vi "Mix signal measurement_1022D.vi"() -> ()   [LabVIEW 2022 SP3]
uses:
  <vilib>/Analysis/baseanly.llb/Mean (DBL).vi
  <vilib>/Utility/file.llb/Write Delimited Spreadsheet (DBL).vi
  <vilib>/Analysis/NI_AALBase.lvlib
panel:
  out "B Frequency(Hz)":sgl=1000.0 min=0.001 max=100000 step=0.001 format="%.3f"
  out "A Frequency(Hz)":sgl=1000.0 min=0.001 max=100000 step=0.001 format="%.3f"
  in  "Differntial  Frequency":dbl=10267.0 format="%#_13g"
  in  "Base Frequency":dbl=10267.0 format="%#_13g"
  in  "Reference Source":u8(ring) items=["External", "Internal", "Internal Sweep", "Channel A"]
  out "B Sum Frequency":dbl=267.77 format="%#_13g"
  in  "B Input Connection (0: Single-Ended)  2":u16(ring)=1 items=["Single-Ended Voltage", "Differential Voltage", "1 MOhm Current Gain", "100 MOhm Current Gain"]
  in  "B harmonic 4":u8=2
  in  "B harmonic 3":u8=3
  in  "B reference Manual Phase 2":dbl=-59.75
  in  "auto phase B 2":bool=TRUE
  in  "B Sample time (s) 2":dbl=0.001 min=0.001 max=100.0 step=0.001
  in  "B Sensitivity  2":u16(ring)=21 items=["1 nV/fA", "2 nV/fA", "5 nV/fA", "10 nV/fA", "20 nV/fA", "50 nV/fA", "100 nV/fA", "200 nV/fA", "500 nV/fA", "1 uV/pA", "2 uV/pA", "5 uV/pA", "10 uV/pA", "20 uV/pA", "50 uV/pA", "100 uV/pA", "200 uV/pA", "500 uV/pA", "1 mV/nA", "2 mV/nA", "5 mV/nA", "10 mV/nA", "20 mV/nA", "50 mV/nA", "100 mV/nA", "200 mV/nA", "500 mV/nA", "1 V/uA"]
  in  "Enable Sync Filter B (open when f<200Hz) 2":bool
  in  "B Time Constant 2":u8(ring)=9 items=["10 us", "30 us", "100 us", "300 us", "1 ms", "3 ms", "10 ms", "30 ms", "100 ms", "300 ms", "1 s", "3 s", "10 s", "30 s", "100 s", "300 s", "1 ks", "3 ks"]
  in  "B Reference Source 2":u8(ring)=1 items=["External", "Internal", "Internal Sweep", "Channel-A"]
  in  "B Low Pass Filter Slope 2":u8(ring)=2 items=["6 dB/oct", "12 dB/oct", "18 db/oct", "24 dB/oct"]
  out "A  Sub Frequency":dbl=267.77 format="%#_13g"
  in  "A Input Connection (0: Single-Ended)  2":u16(ring)=1 items=["Single-Ended Voltage", "Differential Voltage", "1 MOhm Current Gain", "100 MOhm Current Gain"]
  in  "A harmonic 4":u8=2
  in  "A harmonic 3":u8=3
  in  "A reference Manual Phase  2":dbl=-59.75
  in  "auto phase A 2":bool=TRUE
  in  "A Reference Source 2":u8(ring)=1 items=["External", "Internal", "Internal Sweep"]
  in  "A Sample time (s) 2":dbl=0.001 min=0.001 max=100.0 step=0.001
  in  "A Time Constant 2":u8(ring)=9 items=["10 us", "30 us", "100 us", "300 us", "1 ms", "3 ms", "10 ms", "30 ms", "100 ms", "300 ms", "1 s", "3 s", "10 s", "30 s", "100 s", "300 s", "1 ks", "3 ks"]
  in  "Enable Sync Filter A (open when f<200Hz) 2":bool
  in  "A Sensitivity  2":u16(ring)=21 items=["1 nV/fA", "2 nV/fA", "5 nV/fA", "10 nV/fA", "20 nV/fA", "50 nV/fA", "100 nV/fA", "200 nV/fA", "500 nV/fA", "1 uV/pA", "2 uV/pA", "5 uV/pA", "10 uV/pA", "20 uV/pA", "50 uV/pA", "100 uV/pA", "200 uV/pA", "500 uV/pA", "1 mV/nA", "2 mV/nA", "5 mV/nA", "10 mV/nA", "20 mV/nA", "50 mV/nA", "100 mV/nA", "200 mV/nA", "500 mV/nA", "1 V/uA"]
  in  "A Low Pass Filter Slope 2":u8(ring)=2 items=["6 dB/oct", "12 dB/oct", "18 db/oct", "24 dB/oct"]
  in  "LOCKIN2 address":refnum<visa-resource-name>="COM7"
  in  "Series Resistance":string="20kOhm"
  in  "Temperature \n& Field Function":bool=TRUE
  in  "Field Approach":i32(ring) items=["Linear", "NoOvershoot", "Oscillate"]
  in  "F Rate (Oe/s)":dbl=100.0 format="%#_13g"
  in  "Set F (Oe)":dbl format="%#_13g"
  in  "Mode":i32(ring) items=["Persistent", "Driven"]
  in  "Temperature Approach":i32(ring)=1 items=["FastSettle", "NoOvershoot"]
  in  "T  Rate (K/min)":dbl=10.0
  in  "Set  T  (K)":dbl=120.0
  in  "WaitForField":bool=TRUE
  in  "WaitForTemperature":bool=TRUE
  out "Temperature Status":i32(ring) items=["TemperatureUnknown"=0, "Stable"=1, "Tracking"=2, "Near"=5, "Chasing"=6, "Filling"=7, "Standby"=10, "Disabled"=13, "ImpedanceNotFunction"=14, "TempFailure"=15]
  out "Field Status":i32(ring) items=["MagnetUnknown"=0, "StablePersistent"=1, "WarmingSwitch"=2, "CoolingSwitch"=3, "StableDriven"=4, "Iterating"=5, "Charging"=6, "Discharging"=7, "CurrentError"=8, "MagnetFailure"=15]
  out "Field":dbl
  in  "Delay":dbl=5.0
  out "Temperature":dbl
  in  "Remote":bool=TRUE
  in  "IP Address":string="169.254.170.239"
  out "Measuring":bool
  in  "A Low Pass Filter Slope":u8(ring)=2 items=["6 dB/oct", "12 dB/oct", "18 db/oct", "24 dB/oct"]
  in  "B Low Pass Filter Slope":u8(ring)=2 items=["6 dB/oct", "12 dB/oct", "18 db/oct", "24 dB/oct"]
  in  "B Time Constant":u8(ring)=9 items=["10 us", "30 us", "100 us", "300 us", "1 ms", "3 ms", "10 ms", "30 ms", "100 ms", "300 ms", "1 s", "3 s", "10 s", "30 s", "100 s", "300 s", "1 ks", "3 ks"]
  in  "Enable Sync Filter B (open when f<200Hz)":bool
  in  "B Sensitivity":u16(ring)=23 items=["1 nV/fA", "2 nV/fA", "5 nV/fA", "10 nV/fA", "20 nV/fA", "50 nV/fA", "100 nV/fA", "200 nV/fA", "500 nV/fA", "1 uV/pA", "2 uV/pA", "5 uV/pA", "10 uV/pA", "20 uV/pA", "50 uV/pA", "100 uV/pA", "200 uV/pA", "500 uV/pA", "1 mV/nA", "2 mV/nA", "5 mV/nA", "10 mV/nA", "20 mV/nA", "50 mV/nA", "100 mV/nA", "200 mV/nA", "500 mV/nA", "1 V/uA"]
  in  "A Sensitivity":u16(ring)=23 items=["1 nV/fA", "2 nV/fA", "5 nV/fA", "10 nV/fA", "20 nV/fA", "50 nV/fA", "100 nV/fA", "200 nV/fA", "500 nV/fA", "1 uV/pA", "2 uV/pA", "5 uV/pA", "10 uV/pA", "20 uV/pA", "50 uV/pA", "100 uV/pA", "200 uV/pA", "500 uV/pA", "1 mV/nA", "2 mV/nA", "5 mV/nA", "10 mV/nA", "20 mV/nA", "50 mV/nA", "100 mV/nA", "200 mV/nA", "500 mV/nA", "1 V/uA"]
  in  "Enable Sync Filter A (open when f<200Hz)":bool
  in  "A Time Constant":u8(ring)=9 items=["10 us", "30 us", "100 us", "300 us", "1 ms", "3 ms", "10 ms", "30 ms", "100 ms", "300 ms", "1 s", "3 s", "10 s", "30 s", "100 s", "300 s", "1 ks", "3 ks"]
  out "XY Graph 4":cluster{dbl[], dbl[]}(graph)
  in  "Phase B":u16(ring)=9 items=["X", "Y", "R", "Theta", "Frequency", "Noise", "Xh1", "Yh1", "Rh1", "Theta h1", "Xh2", "Yh2", "Rh2", "Theta h2"]
  in  "Parameter B":u16(ring)=8 items=["X", "Y", "R", "Theta", "Frequency", "Noise", "Xh1", "Yh1", "Rh1", "Theta h1", "Xh2", "Yh2", "Rh2", "Theta h2"]
  out "phase B":dbl
  in  "Clear Plot B":bool
  out "XY Graph 3":cluster{dbl[], dbl[]}(graph)
  out "para2 Measurement":dbl=1.49013e-07
  out "XY Graph 2":cluster{dbl[], dbl[]}(graph)
  in  "B Sample time (s)":dbl=0.001 min=0.001 max=100.0 step=0.001
  in  "A Sample time (s)":dbl=0.001 min=0.001 max=100.0 step=0.001
  in  "Phase A":u16(ring)=9 items=["X", "Y", "R", "Theta", "Frequency", "Noise", "Xh1", "Yh1", "Rh1", "Theta h1", "Xh2", "Yh2", "Rh2", "Theta h2"]
  in  "Parameter A":u16(ring)=8 items=["X", "Y", "R", "Theta", "Frequency", "Noise", "Xh1", "Yh1", "Rh1", "Theta h1", "Xh2", "Yh2", "Rh2", "Theta h2"]
  in  "stabilization(S)":dbl=0.1 format="%#_13g"
  in  "B Input Connection (0: Single-Ended)":u16(ring)=1 items=["Single-Ended Voltage", "Differential Voltage", "1 MOhm Current Gain", "100 MOhm Current Gain"]
  in  "B harmonic 1":u8=2
  in  "B harmonic 2":u8=3
  in  "A Input Connection (0: Single-Ended)":u16(ring)=1 items=["Single-Ended Voltage", "Differential Voltage", "1 MOhm Current Gain", "100 MOhm Current Gain"]
  in  "A harmonic 1":u8=2
  in  "A harmonic 2":u8=3
  in  "A Reference Source":u8(ring)=1 items=["External", "Internal", "Internal Sweep"]
  out "phase A":dbl
  out "loop run":i32
  in  "loop #":i32=1
  in  "Save data or not":bool=TRUE
  in  "path (folder + filename)":string="G:\\My Drive\\Opticool\\Measurement\\NLH\\Signal Mixing\\TaI18_test"
  in  "Clear Plot A":bool
  out "XY Graph":cluster{dbl[], dbl[]}(graph)={[0.18, 0.16, 0.14, 0.12000000000000001, 0.1], [3.3030160227288526e-06, 3.321717991170714e-05, 7.096266610655447e-06, 1.857138617731224e-05, 2.1320792974836174e-05]}
  out "para1 Measurement":dbl=1.49013e-07
  out "Sine voltage":dbl format="%#_13g"
  in  "GATE STEP(mv)":i32=20
  in  "Sine Low Value (default 0V)":dbl=0.1
  in  "Sine High Value (0.001-5V)":dbl=1.0
  in  "lockin waiting (s)":dbl=0.1 format="%#_13g"
  in  "LOCKIN1 address":refnum<visa-resource-name>="COM3"
  # "Lock-in 1 Setting (Input)"
  # "Channel A"
  # "Channel B"
  # "Lock-in 2 Setting (Measure)"
  # "Channel A"
  # "Channel B"
  # "Mesurement"
  # "Sine Sweep Setting"
  # "Temprature and Field Setting"
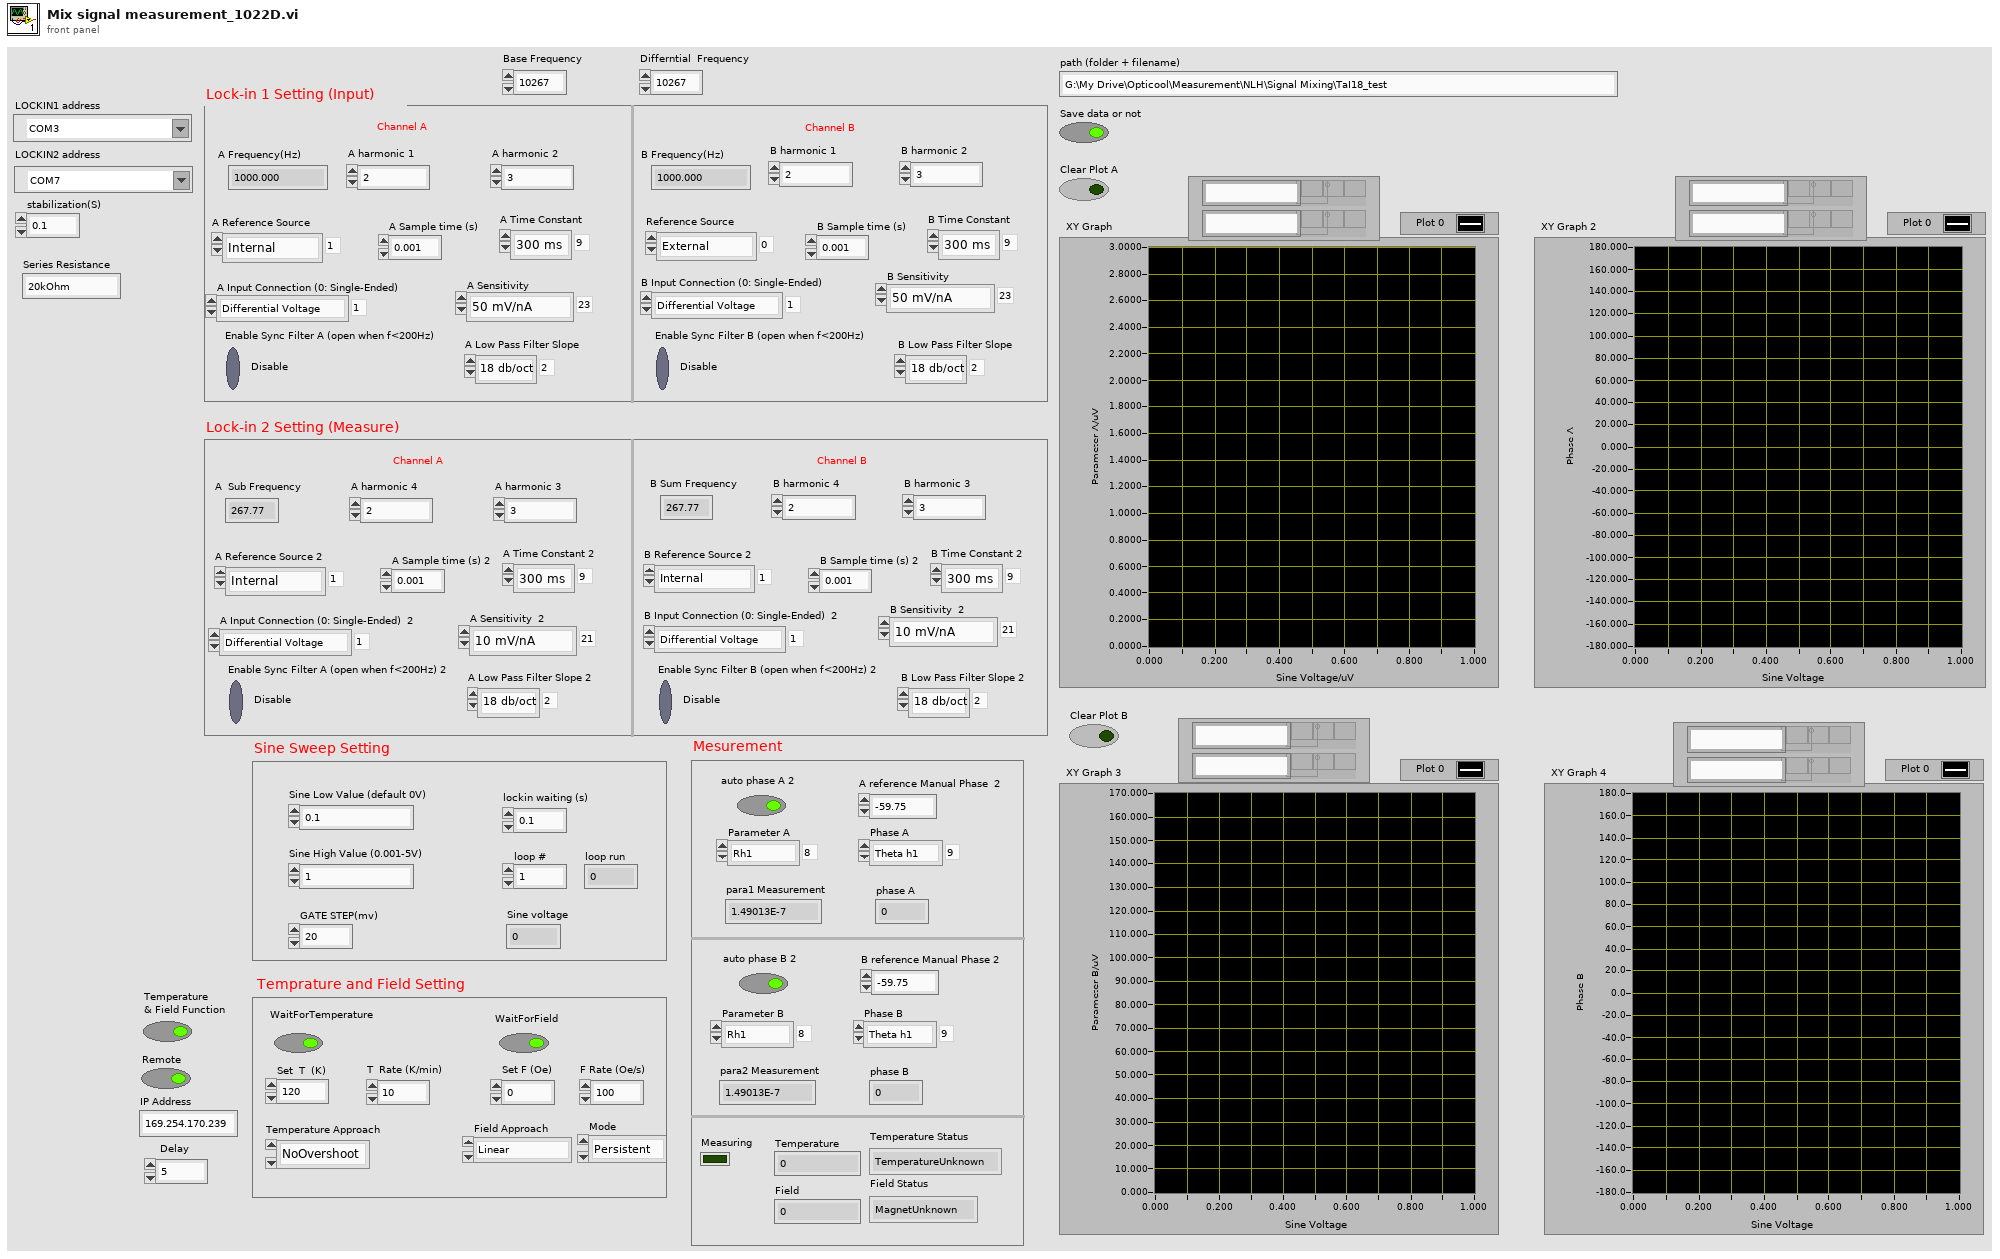
[diagram p1: front panel]
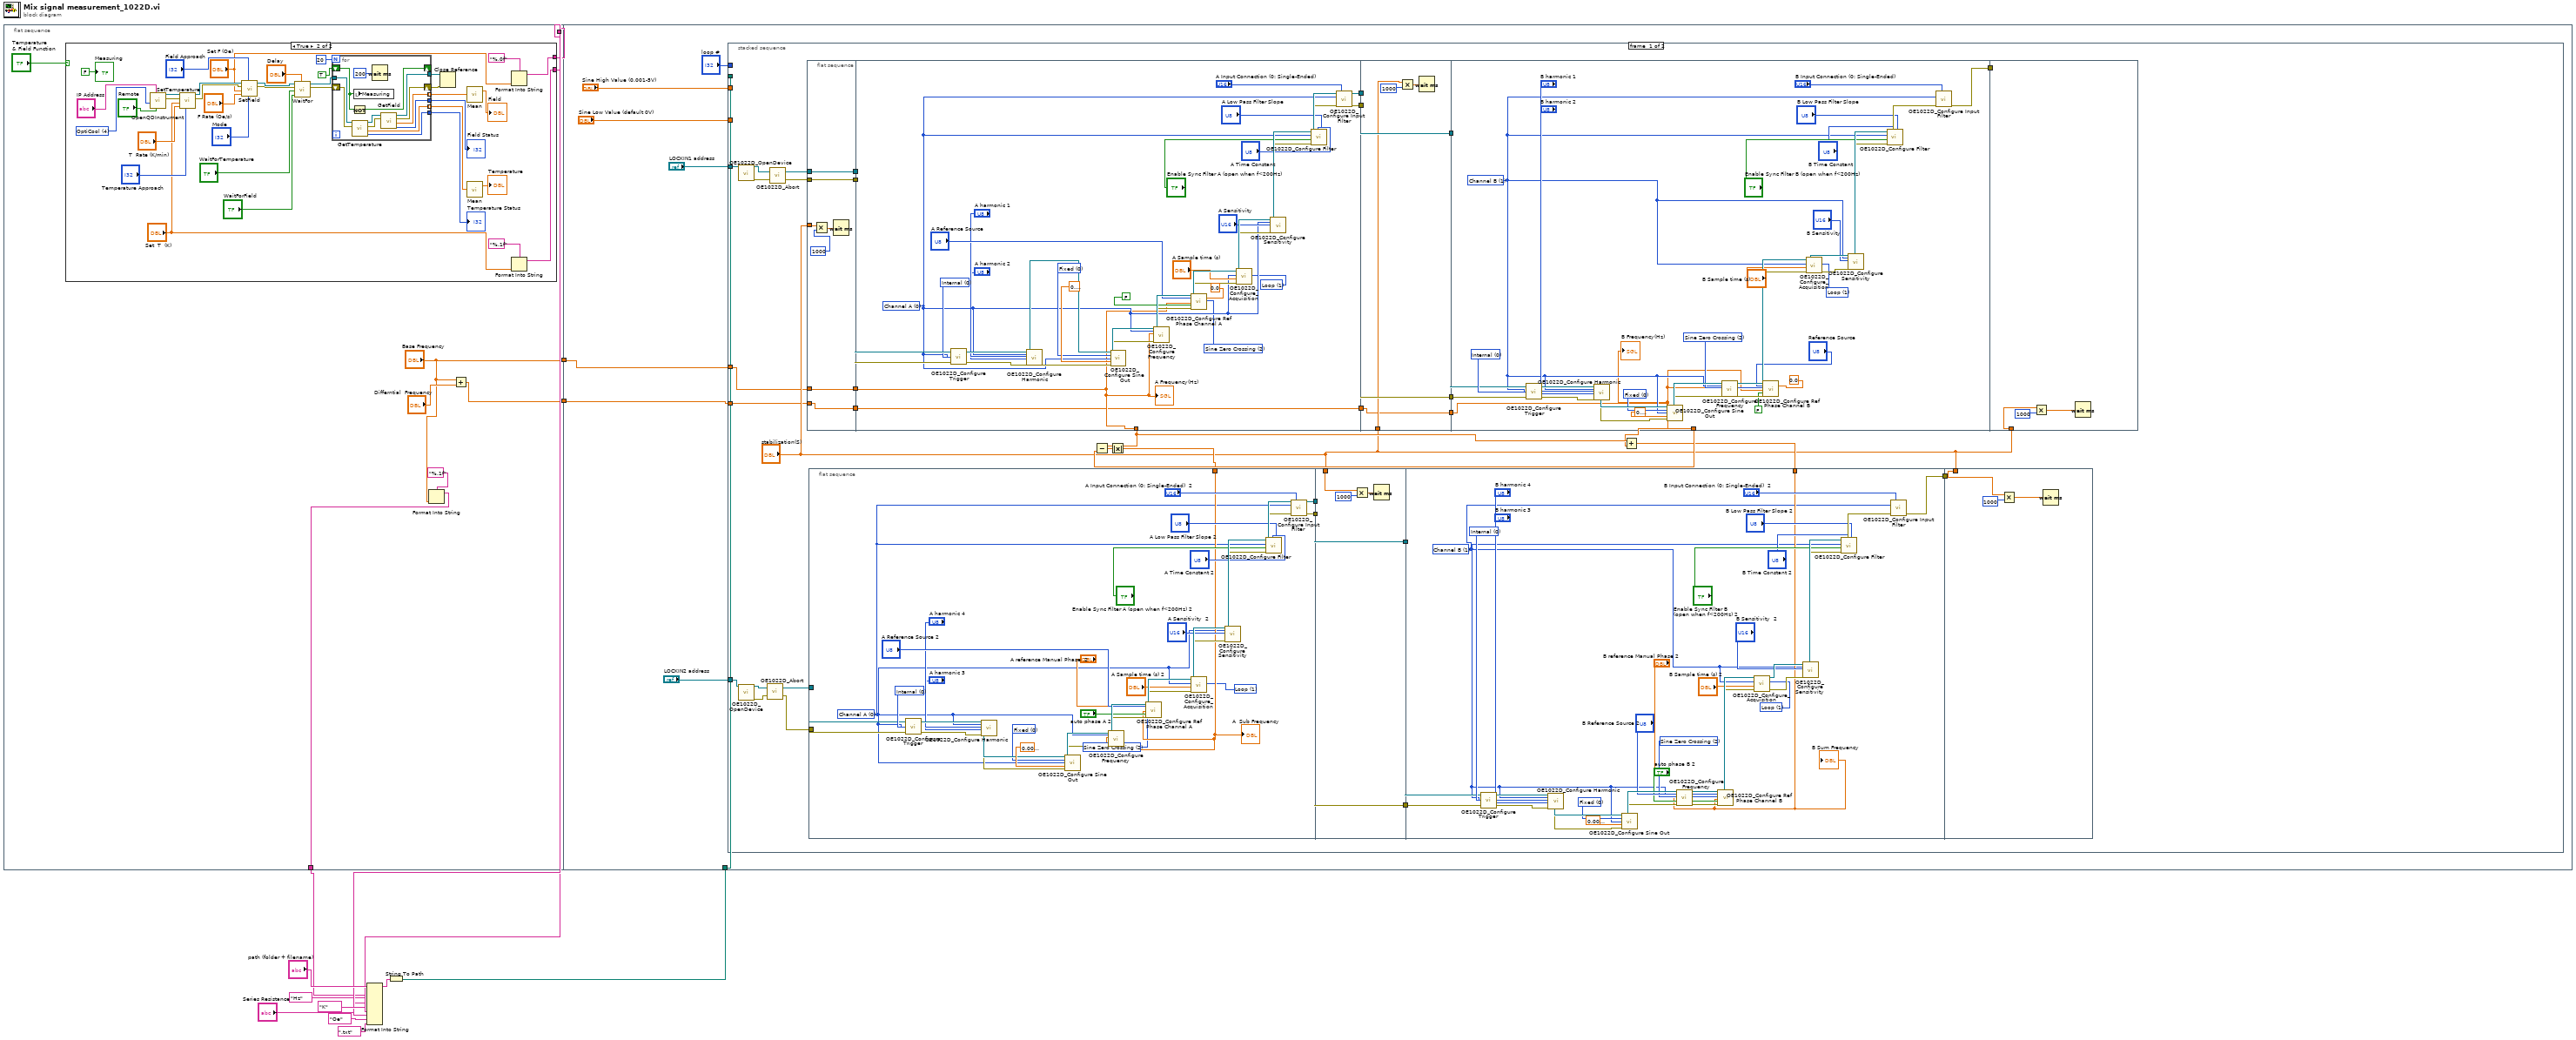
[diagram p0: block diagram]
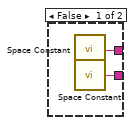
[diagram p2: hidden frame]
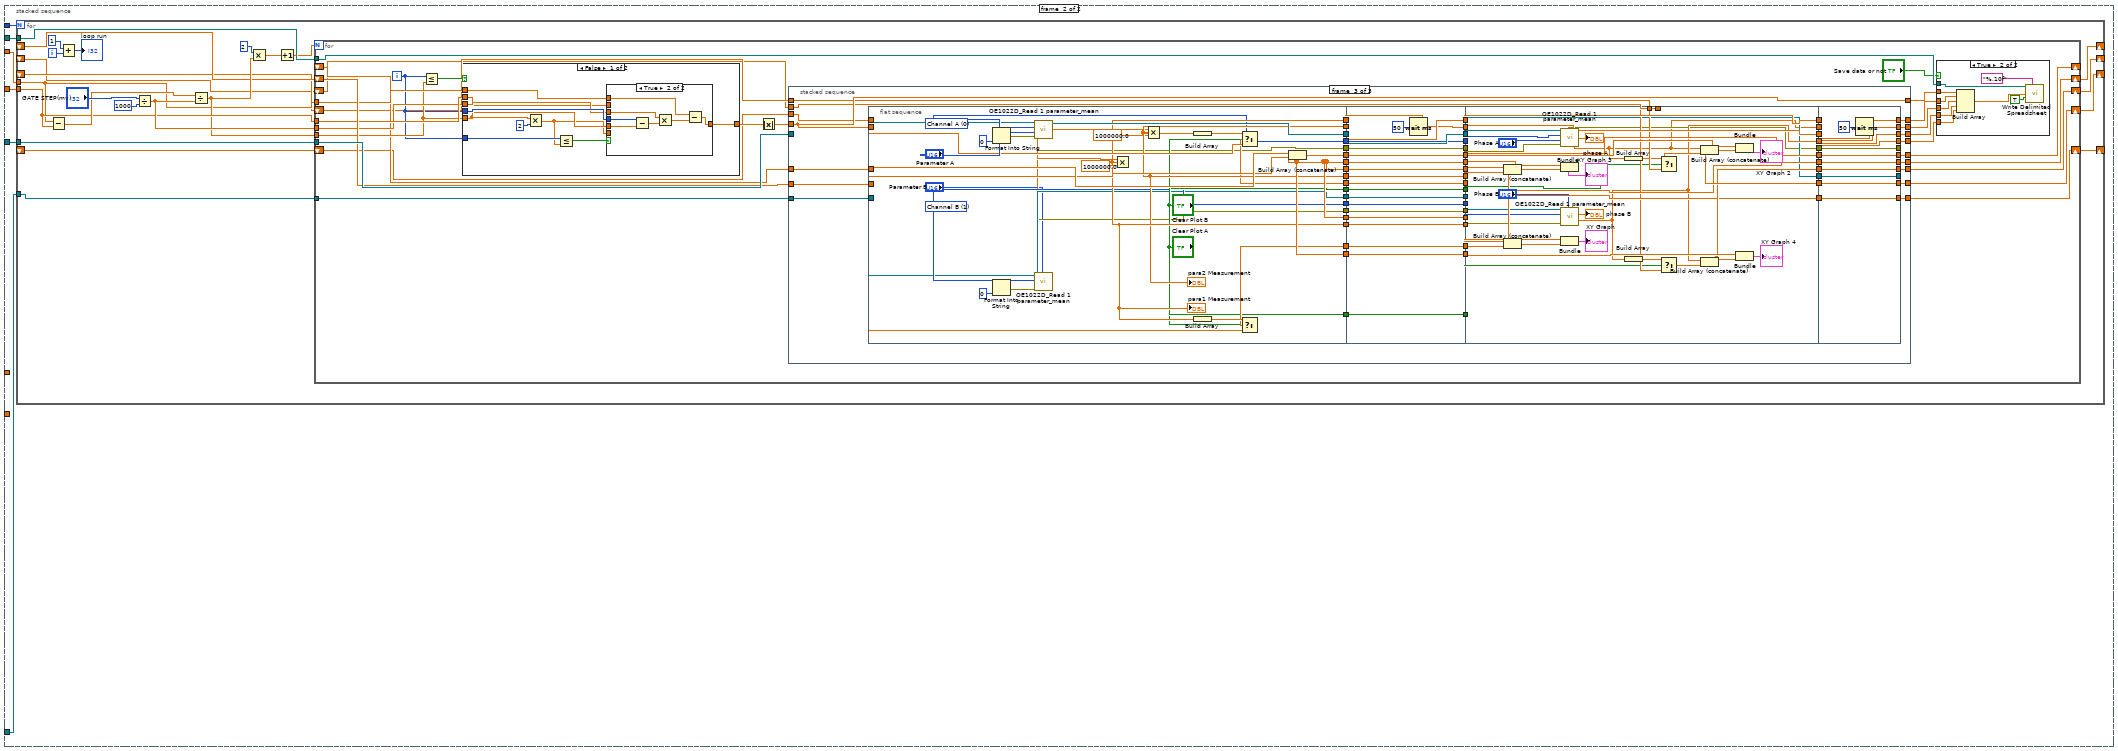
[diagram p3: hidden frame]
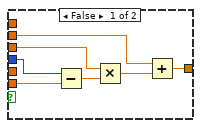
[diagram p5: hidden frame]
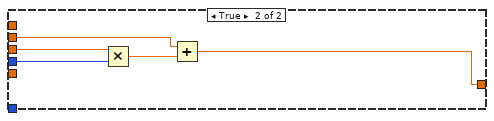
[diagram p6: hidden frame]
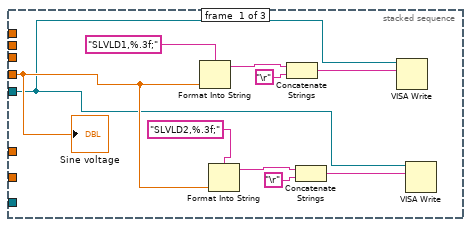
[diagram p7: hidden frame]
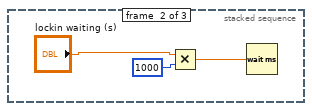
[diagram p8: hidden frame]
diagram:
  n1 = flat-sequence {
    tunnel: [w21] -> w6
    tunnel: [w20] -> w10
    tunnel: [w16] -> w4
    tunnel: ["Base Frequency"] -> w3
    tunnel: [w14] -> w2
    tunnel: w13 -> [w77]
    tunnel: w4 -> [w74]
    tunnel: w3 -> [w73]
    frame #0 {
      n2 = case shown="True" "Temperature \n& Field Function" {
        tunnel: [w23 w25] -> w21
        tunnel: [w22 w24] -> w20
        frame False {
          n3 = call <vilib>:"Space Constant.vi"() -> ("String"=w22:string)
          n4 = call <vilib>:"Space Constant.vi"() -> ("String"=w23:string)
        }
        frame True {
          w50 = 4 items=["PPMS", "VersaLab", "DynaCool", "SVSM", "OptiCool"] ("InstrumentType")
          n5 = call "OpenQDInstrument.vi"("Remote"="Remote", "IP Address"="IP Address", "InstrumentType"=w50) -> ("error out"=w37:errorcluster, "Instrument Ref"=w38:refnum<k24>)  [unwired: 5 in]
          n6 = call "SetTemperature.vi"("Approach"="Temperature Approach", "Rate"="T  Rate (K/min)", "Temperature"="Set  T  (K)", "error in (no error)"=w37, "Instrument Ref In"=w38) -> ("error out"=w56:errorcluster, "Instrument Ref Out"=w55:refnum<k24>)  [unwired: 2 in, 1 out]
          n7 = call "SetField.vi"("Mode"="Mode", "Approach"="Field Approach", "Rate"="F Rate (Oe/s)", "Field"="Set F (Oe)", "error in (no error)"=w56, "Instrument Ref In"=w55) -> ("error out"=w33:errorcluster, "Instrument Ref Out"=w34:refnum<k24>)  [unwired: 1 in, 1 out]
          n8 = call "WaitFor.vi"("Delay"="Delay", "Wait For Field"="WaitForField", "Wait For Temperature"="WaitForTemperature", "error in (no error)"=w33, "Instrument Ref In"=w34) -> ("error out"=w49:errorcluster, "Instrument Ref Out"=w45:refnum<k24>)  [unwired: 5 in]
          n9 = for {
            N: 20 -> [_]
            shift-right: [w72] -> _
            shift-left: TRUE -> [w70]
            shift-right: [w67] -> w35
            shift-left: w49 -> [w69]
            tunnel: w45 -> [w66]
            tunnel: [w64] -> w36
            tunnel: [w61] -> w44
            tunnel: [w60] -> w43
            tunnel: [w62] -> w41 mode=indexing
            tunnel: [w63] -> w42 mode=indexing
            n10 = Not(x=w70) -> (.not. x?=w72:bool)
            n11 = call "GetTemperature.vi"("error in (no error)"=w69, "Instrument Ref In"=w66) -> ("Temperature\nStatus"=w60:i32, "Temperature"=w63:dbl, "error out"=w68:errorcluster, "Instrument Ref Out"=w65:refnum<k24>)  [unwired: 3 in, 1 out]
            n12 = local write "Measuring"(w70) -> ()
            n13 = Wait (ms)(milliseconds to wait=u32 200) -> ()  [unwired: 1 out]
            n14 = call "GetField.vi"("error in (no error)"=w68, "Instrument Ref In"=w65) -> ("Field\nStatus"=w61:i32, "Field"=w62:dbl, "error out"=w67:errorcluster, "Instrument Ref Out"=w64:refnum<k24>)  [unwired: 3 in, 1 out]
          }
          "Field Status" <- w44
          "Temperature Status" <- w43
          n15 = Close Reference(reference=w36, error in (no error)=w35) -> ()  [unwired: 1 out]
          n16 = call-poly <vilib>:"Mean.vi"("X"=w41) -> ("mean"=→"Field":dbl)  [unwired: 1 out]
          n17 = call-poly <vilib>:"Mean.vi"("X"=w42) -> ("mean"=→"Temperature":dbl)  [unwired: 1 out]
          n18 = Format Into String(format string="%.0f", "Set F (Oe)") -> (resulting string=w24:string)  [unwired: 2 in, 1 out]
          n19 = Format Into String(format string="%.1f", "Set  T  (K)") -> (resulting string=w25:string)  [unwired: 2 in, 1 out]
          "Measuring" <- FALSE
        }
      }
      n20 = Format Into String(format string="%.1f", "Base Frequency") -> (resulting string=w14:string)  [unwired: 2 in, 1 out]
      n21 = Add(x="Base Frequency", y="Differntial  Frequency") -> (x+y=w16:dbl)
    }
    frame #1 {
      n22 = stacked-sequence {
        tunnel: "LOCKIN1 address" -> [w106 w293]
        tunnel: "Sine High Value (0.001-5V)" -> [_ w291]
        tunnel: "Sine Low Value (default 0V)" -> [_ w292]
        tunnel: w77 -> [_ w290]
        tunnel: "loop #" -> [_ w289]
        tunnel: "LOCKIN2 address" -> [w102 w288]
        tunnel: w73 -> [w86 _]
        tunnel: w74 -> [w84 _]
        frame #0 {
          n23 = call <instrlib>:"OE1022D_OpenDevice.vi"("VISA resource name"=w106) -> ("VISA资源名称输出"=w105:refnum<visa-resource-name>, "错误输出"=w107:errorcluster)  [unwired: 17 in]
          n24 = call <instrlib>:"OE1022D_OpenDevice.vi"("VISA resource name"=w102) -> ("VISA资源名称输出"=w103:refnum<visa-resource-name>, "错误输出"=w104:errorcluster)  [unwired: 17 in]
          n25 = call <instrlib>:"OE1022D_Abort.vi"("error in (no error)"=w104, "VISA resource name"=w103) -> ("error out"=w95:errorcluster, "VISA resource name out"=w96:refnum<visa-resource-name>)
          n26 = call <instrlib>:"OE1022D_Abort.vi"("error in (no error)"=w107, "VISA resource name"=w105) -> ("error out"=w112:errorcluster, "VISA resource name out"=w113:refnum<visa-resource-name>)
          n27 = flat-sequence {
            tunnel: w112 -> [w202]
            tunnel: w113 -> [w203]
            tunnel: [w203] -> w89
            tunnel: [w202] -> w88
            tunnel: "stabilization(S)" -> [w199]
            tunnel: w86 -> [w198]
            tunnel: [w198] -> w85
            tunnel: w84 -> [w197]
            tunnel: [w197] -> w83
            tunnel: [w232] -> w111
            tunnel: [w221] -> w109
            tunnel: [w205] -> w93
            tunnel: w89 -> [w242]
            tunnel: w88 -> [w241]
            tunnel: w85 -> [w205]
            tunnel: w83 -> [w204]
            tunnel: [w204] -> w82
            tunnel: w111 -> [w248]
            tunnel: [w248] -> w110
            tunnel: w109 -> [w247]
            tunnel: [w247] -> w108
            tunnel: "stabilization(S)" -> [w244]
            tunnel: w82 -> [w243]
            tunnel: [w243] -> w81
            tunnel: w110 -> [w270]
            tunnel: [w269] -> w114
            tunnel: w108 -> [w268]
            tunnel: [w249] -> w92
            tunnel: w81 -> [w249]
            tunnel: w114 -> [_]
            tunnel: "stabilization(S)" -> [w285]
            frame #0 {
              n28 = Multiply(x=w199, y=1000) -> (x*y=w201:dbl)
              n29 = Wait (ms)(milliseconds to wait=w201) -> ()  [unwired: 1 out]
            }
            frame #1 {
              w206 = u8 2 items=["TTL Pos", "TTL Neg", "Sine Zero Crossing"] ("External Ref Trigger")
              w207 = u8 1 items=["Single", "Loop"] ("Sample Mode (Single/Loop)")
              w220 = u8 0 items=["Fixed", "Linear", "Log"] ("SineOut Mode")
              w222 = u16 0 items=["Internal", "External"] ("Trigger Source (0: Internal)")
              w208 = u8 0 items=["Channel A", "Channel B"] ("OE1022D A/B")
              n30 = call <instrlib>:"OE1022D_Configure Trigger.vi"("Trigger Source (0: Internal)"=w222, "error in (no error)   2"=w241, "OE1022D A/B"=w208, "VISA resource name   2"=w242) -> ("error out   2"=w235:errorcluster, "VISA resource name out   2"=w236:refnum<visa-resource-name>)
              n31 = call <instrlib>:"OE1022D_Configure Harmonic.vi"("VISA resource name"=w236, "OE1022D A/B"=w208, "Harmonic 1"="A harmonic 1", "Harmonic 2"="A harmonic 2", "error in (no error)"=w235) -> ("VISA resource name out"=w234:refnum<visa-resource-name>, "error out"=w233:errorcluster)  [unwired: 13 in]
              n32 = call <instrlib>:"OE1022D_Configure Sine Out.vi"("VISA resource name"=w234, "SineOut Mode"=w220, "OE1022D A/B"=w208, "Sine Output Amplitude (V)"=sgl 0.1, "error in (no error)"=w233) -> ("VISA resource name out"=w239:refnum<visa-resource-name>, "error out"=w238:errorcluster)  [unwired: 9 in]
              n33 = call <instrlib>:"OE1022D_Configure Frequency.vi"("VISA resource name"=w239, "OE1022D A/B"=w208, "Internal Frequency(Hz)"=w205, "error in (no error)"=w238) -> ("VISA resource name out"=w231:refnum<visa-resource-name>, "error out"=w228:errorcluster)  [unwired: 14 in]
              n34 = call <instrlib>:"OE1022D_Configure Ref Phase Channel A.vi"("VISA resource name"=w231, "Reference Source"="A Reference Source", "External Ref Trigger"=w206, "Internal Frequency(Hz)"=w205, "Auto Phase (T: Enabled)"=FALSE ("auto phase A"), "error in (no error)"=w228, "Manual Phase  (degree)"=0.0 ("A reference Manual Phase")) -> ("VISA resource name out"=w230:refnum<visa-resource-name>, "error out"=w229:errorcluster)  [unwired: 11 in]
              n35 = call <instrlib>:"OE1022D_Configure_Acquisition.vi"("VISA resource name"=w230, "OE1022D A/B"=w208, "Sample time (s)"="A Sample time (s)", "error in (no error)"=w229, "Sample Mode (Single/Loop)"=w207) -> ("VISA resource name out"=w214:refnum<visa-resource-name>, "error out"=w213:errorcluster)  [unwired: 3 in]
              n36 = call <instrlib>:"OE1022D_Configure Sensitivity.vi"("VISA resource name"=w214, "OE1022D A/B"=w208, "Sensitivity"="A Sensitivity", "error in (no error)"=w213) -> ("VISA resource name out"=w218:refnum<visa-resource-name>, "error out"=w217:errorcluster)  [unwired: 14 in]
              n37 = call <instrlib>:"OE1022D_Configure Filter.vi"("Low Pass Filter Slope (1: 12dB/oct)"="A Low Pass Filter Slope", "Time Constant (8: 100ms)"="A Time Constant", "error in (no error)"=w217, "Enable Sync Filter (F: Disable)"="Enable Sync Filter A (open when f<200Hz)", "OE1022D A/B"=w208, "VISA resource name"=w218) -> ("error out"=w215:errorcluster, "VISA resource name out"=w216:refnum<visa-resource-name>)  [unwired: 4 in]
              n38 = call <instrlib>:"OE1022D_Configure Input Filter.vi"("VISA resource name"=w216, "Input Source"="A Input Connection (0: Single-Ended)", "OE1022D A/B"=w208, "error in (no error)"=w215) -> ("VISA resource name out"=w221:refnum<visa-resource-name>, "error out"=w232:errorcluster)  [unwired: 10 in]
              "A Frequency(Hz)" <- w205
            }
            frame #2 {
              n39 = Multiply(x=w244, y=1000) -> (x*y=w246:dbl)
              n40 = Wait (ms)(milliseconds to wait=w246) -> ()  [unwired: 1 out]
            }
            frame #3 {
              w251 = u8 1 items=["Single", "Loop"] ("Sample Mode (Single/Loop)")
              w254 = u8 2 items=["TTL Pos", "TTL Neg", "Sine Zero Crossing"] ("External Ref Trigger")
              w265 = u8 0 items=["Fixed", "Linear", "Log"] ("SineOut Mode")
              w271 = u16 0 items=["Internal", "External"] ("Trigger Source (0: Internal)")
              w252 = u8 1 items=["Channel A", "Channel B"] ("OE1022D A/B")
              n41 = call <instrlib>:"OE1022D_Configure Trigger.vi"("Trigger Source (0: Internal)"=w271, "error in (no error)   2"=w270, "OE1022D A/B"=w252, "VISA resource name   2"=w268) -> ("error out   2"=w280:errorcluster, "VISA resource name out   2"=w281:refnum<visa-resource-name>)
              n42 = call <instrlib>:"OE1022D_Configure Harmonic.vi"("VISA resource name"=w281, "OE1022D A/B"=w252, "Harmonic 1"="B harmonic 1", "Harmonic 2"="B harmonic 2", "error in (no error)"=w280) -> ("VISA resource name out"=w279:refnum<visa-resource-name>, "error out"=w278:errorcluster)  [unwired: 13 in]
              n43 = call <instrlib>:"OE1022D_Configure Sine Out.vi"("VISA resource name"=w279, "SineOut Mode"=w265, "OE1022D A/B"=w252, "Sine Output Amplitude (V)"=sgl 0.1, "error in (no error)"=w278) -> ("VISA resource name out"=w283:refnum<visa-resource-name>, "error out"=w282:errorcluster)  [unwired: 9 in]
              n44 = call <instrlib>:"OE1022D_Configure Frequency.vi"("VISA resource name"=w283, "OE1022D A/B"=w252, "Internal Frequency(Hz)"=w249, "error in (no error)"=w282) -> ("VISA resource name out"=w277:refnum<visa-resource-name>, "error out"=w274:errorcluster)  [unwired: 14 in]
              n45 = call <instrlib>:"OE1022D_Configure Ref Phase Channel B.vi"("VISA resource name"=w277, "Reference Source"="Reference Source", "External Ref Trigger"=w254, "Internal Frequency(Hz)"=w249, "Auto Phase (T: Enabled)"=FALSE ("auto phase B"), "error in (no error)"=w274, "Manual Phase  (degree)"=0.0 ("B reference Manual Phase")) -> ("VISA resource name out"=w276:refnum<visa-resource-name>, "error out"=w275:errorcluster)  [unwired: 11 in]
              n46 = call <instrlib>:"OE1022D_Configure_Acquisition.vi"("VISA resource name"=w276, "OE1022D A/B"=w252, "Sample time (s)"="B Sample time (s)", "error in (no error)"=w275, "Sample Mode (Single/Loop)"=w251) -> ("VISA resource name out"=w258:refnum<visa-resource-name>, "error out"=w259:errorcluster)  [unwired: 3 in]
              n47 = call <instrlib>:"OE1022D_Configure Sensitivity.vi"("VISA resource name"=w258, "OE1022D A/B"=w252, "Sensitivity"="B Sensitivity", "error in (no error)"=w259) -> ("VISA resource name out"=w262:refnum<visa-resource-name>, "error out"=w261:errorcluster)  [unwired: 14 in]
              n48 = call <instrlib>:"OE1022D_Configure Filter.vi"("Low Pass Filter Slope (1: 12dB/oct)"="B Low Pass Filter Slope", "Time Constant (8: 100ms)"="B Time Constant", "error in (no error)"=w261, "Enable Sync Filter (F: Disable)"="Enable Sync Filter B (open when f<200Hz)", "OE1022D A/B"=w252, "VISA resource name"=w262) -> ("error out"=w260:errorcluster)  [unwired: 4 in, 1 out]
              n49 = call <instrlib>:"OE1022D_Configure Input Filter.vi"("Input Source"="B Input Connection (0: Single-Ended)", "OE1022D A/B"=w252, "error in (no error)"=w260) -> ("error out"=w269:errorcluster)  [unwired: 11 in, 1 out]
              "B Frequency(Hz)" <- w249
            }
            frame #4 {
              n50 = Multiply(x=w285, y=1000) -> (x*y=w287:dbl)
              n51 = Wait (ms)(milliseconds to wait=w287) -> ()  [unwired: 1 out]
            }
          }
          n52 = flat-sequence {
            tunnel: [w144] -> w101
            tunnel: [w133] -> w100
            tunnel: w96 -> [w120]
            tunnel: w95 -> [w119]
            tunnel: w91 -> [w118]
            tunnel: w101 -> [w157]
            tunnel: [w157] -> w99
            tunnel: w100 -> [w156]
            tunnel: [w156] -> w98
            tunnel: "stabilization(S)" -> [w153]
            tunnel: w99 -> [w178]
            tunnel: [w177] -> w97
            tunnel: w98 -> [w176]
            tunnel: w90 -> [w160]
            tunnel: w97 -> [_]
            tunnel: "stabilization(S)" -> [w194]
            frame #0 {
              w115 = u8 2 items=["TTL Pos", "TTL Neg", "Sine Zero Crossing"] ("External Ref Trigger")
              w116 = u8 1 items=["Single", "Loop"] ("Sample Mode (Single/Loop)")
              w132 = u8 0 items=["Fixed", "Linear", "Log"] ("SineOut Mode")
              w134 = u16 0 items=["Internal", "External"] ("Trigger Source (0: Internal)")
              w117 = u8 0 items=["Channel A", "Channel B"] ("OE1022D A/B")
              n53 = call <instrlib>:"OE1022D_Configure Trigger.vi"("Trigger Source (0: Internal)"=w134, "error in (no error)   2"=w119, "OE1022D A/B"=w117, "VISA resource name   2"=w120) -> ("error out   2"=w147:errorcluster, "VISA resource name out   2"=w148:refnum<visa-resource-name>)
              n54 = call <instrlib>:"OE1022D_Configure Harmonic.vi"("VISA resource name"=w148, "OE1022D A/B"=w117, "Harmonic 1"="A harmonic 4", "Harmonic 2"="A harmonic 3", "error in (no error)"=w147) -> ("VISA resource name out"=w146:refnum<visa-resource-name>, "error out"=w145:errorcluster)  [unwired: 13 in]
              n55 = call <instrlib>:"OE1022D_Configure Sine Out.vi"("VISA resource name"=w146, "SineOut Mode"=w132, "OE1022D A/B"=w117, "Sine Output Amplitude (V)"=sgl 0.01, "error in (no error)"=w145) -> ("VISA resource name out"=w151:refnum<visa-resource-name>, "error out"=w150:errorcluster)  [unwired: 9 in]
              n56 = call <instrlib>:"OE1022D_Configure Frequency.vi"("VISA resource name"=w151, "OE1022D A/B"=w117, "Internal Frequency(Hz)"=w118, "error in (no error)"=w150) -> ("VISA resource name out"=w143:refnum<visa-resource-name>, "error out"=w140:errorcluster)  [unwired: 14 in]
              n57 = call <instrlib>:"OE1022D_Configure Ref Phase Channel A.vi"("VISA resource name"=w143, "Reference Source"="A Reference Source 2", "External Ref Trigger"=w115, "Internal Frequency(Hz)"=w118, "Auto Phase (T: Enabled)"="auto phase A 2", "error in (no error)"=w140, "Manual Phase  (degree)"="A reference Manual Phase  2") -> ("VISA resource name out"=w142:refnum<visa-resource-name>, "error out"=w141:errorcluster)  [unwired: 11 in]
              n58 = call <instrlib>:"OE1022D_Configure_Acquisition.vi"("VISA resource name"=w142, "OE1022D A/B"=w117, "Sample time (s)"="A Sample time (s) 2", "error in (no error)"=w141, "Sample Mode (Single/Loop)"=w116) -> ("VISA resource name out"=w126:refnum<visa-resource-name>, "error out"=w125:errorcluster)  [unwired: 3 in]
              n59 = call <instrlib>:"OE1022D_Configure Sensitivity.vi"("VISA resource name"=w126, "OE1022D A/B"=w117, "Sensitivity"="A Sensitivity  2", "error in (no error)"=w125) -> ("VISA resource name out"=w130:refnum<visa-resource-name>, "error out"=w129:errorcluster)  [unwired: 14 in]
              n60 = call <instrlib>:"OE1022D_Configure Filter.vi"("Low Pass Filter Slope (1: 12dB/oct)"="A Low Pass Filter Slope 2", "Time Constant (8: 100ms)"="A Time Constant 2", "error in (no error)"=w129, "Enable Sync Filter (F: Disable)"="Enable Sync Filter A (open when f<200Hz) 2", "OE1022D A/B"=w117, "VISA resource name"=w130) -> ("error out"=w127:errorcluster, "VISA resource name out"=w128:refnum<visa-resource-name>)  [unwired: 4 in]
              n61 = call <instrlib>:"OE1022D_Configure Input Filter.vi"("VISA resource name"=w128, "Input Source"="A Input Connection (0: Single-Ended)  2", "OE1022D A/B"=w117, "error in (no error)"=w127) -> ("VISA resource name out"=w133:refnum<visa-resource-name>, "error out"=w144:errorcluster)  [unwired: 10 in]
              "A  Sub Frequency" <- w118
            }
            frame #1 {
              n62 = Multiply(x=w153, y=1000) -> (x*y=w155:dbl)
              n63 = Wait (ms)(milliseconds to wait=w155) -> ()  [unwired: 1 out]
            }
            frame #2 {
              w158 = u8 1 items=["Single", "Loop"] ("Sample Mode (Single/Loop)")
              w162 = u8 2 items=["TTL Pos", "TTL Neg", "Sine Zero Crossing"] ("External Ref Trigger")
              w173 = u8 0 items=["Fixed", "Linear", "Log"] ("SineOut Mode")
              w179 = u16 0 items=["Internal", "External"] ("Trigger Source (0: Internal)")
              w159 = u8 1 items=["Channel A", "Channel B"] ("OE1022D A/B")
              n64 = call <instrlib>:"OE1022D_Configure Trigger.vi"("Trigger Source (0: Internal)"=w179, "error in (no error)   2"=w178, "OE1022D A/B"=w159, "VISA resource name   2"=w176) -> ("error out   2"=w189:errorcluster, "VISA resource name out   2"=w190:refnum<visa-resource-name>)
              n65 = call <instrlib>:"OE1022D_Configure Harmonic.vi"("VISA resource name"=w190, "OE1022D A/B"=w159, "Harmonic 1"="B harmonic 4", "Harmonic 2"="B harmonic 3", "error in (no error)"=w189) -> ("VISA resource name out"=w188:refnum<visa-resource-name>, "error out"=w187:errorcluster)  [unwired: 13 in]
              n66 = call <instrlib>:"OE1022D_Configure Sine Out.vi"("VISA resource name"=w188, "SineOut Mode"=w173, "OE1022D A/B"=w159, "Sine Output Amplitude (V)"=sgl 0.01, "error in (no error)"=w187) -> ("VISA resource name out"=w192:refnum<visa-resource-name>, "error out"=w191:errorcluster)  [unwired: 9 in]
              n67 = call <instrlib>:"OE1022D_Configure Frequency.vi"("VISA resource name"=w192, "OE1022D A/B"=w159, "Internal Frequency(Hz)"=w160, "error in (no error)"=w191) -> ("VISA resource name out"=w186:refnum<visa-resource-name>, "error out"=w183:errorcluster)  [unwired: 14 in]
              n68 = call <instrlib>:"OE1022D_Configure Ref Phase Channel B.vi"("VISA resource name"=w186, "Reference Source"="B Reference Source 2", "External Ref Trigger"=w162, "Internal Frequency(Hz)"=w160, "Auto Phase (T: Enabled)"="auto phase B 2", "error in (no error)"=w183, "Manual Phase  (degree)"="B reference Manual Phase 2") -> ("VISA resource name out"=w185:refnum<visa-resource-name>, "error out"=w184:errorcluster)  [unwired: 11 in]
              n69 = call <instrlib>:"OE1022D_Configure_Acquisition.vi"("VISA resource name"=w185, "OE1022D A/B"=w159, "Sample time (s)"="B Sample time (s) 2", "error in (no error)"=w184, "Sample Mode (Single/Loop)"=w158) -> ("VISA resource name out"=w166:refnum<visa-resource-name>, "error out"=w167:errorcluster)  [unwired: 3 in]
              n70 = call <instrlib>:"OE1022D_Configure Sensitivity.vi"("VISA resource name"=w166, "OE1022D A/B"=w159, "Sensitivity"="B Sensitivity  2", "error in (no error)"=w167) -> ("VISA resource name out"=w170:refnum<visa-resource-name>, "error out"=w169:errorcluster)  [unwired: 14 in]
              n71 = call <instrlib>:"OE1022D_Configure Filter.vi"("Low Pass Filter Slope (1: 12dB/oct)"="B Low Pass Filter Slope 2", "Time Constant (8: 100ms)"="B Time Constant 2", "error in (no error)"=w169, "Enable Sync Filter (F: Disable)"="Enable Sync Filter B (open when f<200Hz) 2", "OE1022D A/B"=w159, "VISA resource name"=w170) -> ("error out"=w168:errorcluster)  [unwired: 4 in, 1 out]
              n72 = call <instrlib>:"OE1022D_Configure Input Filter.vi"("Input Source"="B Input Connection (0: Single-Ended)  2", "OE1022D A/B"=w159, "error in (no error)"=w168) -> ("error out"=w177:errorcluster)  [unwired: 11 in, 1 out]
              "B Sum Frequency" <- w160
            }
            frame #3 {
              n73 = Multiply(x=w194, y=1000) -> (x*y=w196:dbl)
              n74 = Wait (ms)(milliseconds to wait=w196) -> ()  [unwired: 1 out]
            }
          }
          n75 = Subtract(x=w93, y=w92) -> (x-y=w94:dbl)
          n76 = Absolute Value(x=w94) -> (abs(x)=w91:dbl)
          n77 = Add(x=w93, y=w92) -> (x+y=w90:dbl)
        }
        frame #1 {
          n78 = for {
            N: w289 -> [_]
            tunnel: w293 -> [w317]
            tunnel: w292 -> [w311]
            tunnel: w291 -> [w301]
            tunnel: w290 -> [w310]
            shift-right: [w306] -> _
            shift-left: _ -> [w305]
            shift-right: [w300] -> _
            shift-left: _ -> [w299]
            shift-right: [w298] -> _
            shift-left: _ -> [w297]
            shift-right: [w296] -> _
            shift-left: _ -> [w295]
            tunnel: w288 -> [w294]
            i -> [w303]
            n79 = Subtract(x=w301, y=w311) -> (x-y=w313:dbl)
            n80 = Add(x=1, y=w303) -> (x+y=→"loop run":i32)
            n81 = Divide(x="GATE STEP(mv)", y=1000) -> (x/y=w312:dbl)
            n82 = Divide(x=w313, y=w312) -> (x/y=w309:dbl)
            n83 = Multiply(x=2, y=w309) -> (x*y=w308:dbl)
            n84 = Increment(x=w308) -> (x+1=w307:dbl)
            n85 = for {
              N: w307 -> [_]
              tunnel: w317 -> [w344]
              tunnel: w312 -> [w340]
              shift-right: [w326] -> w306
              shift-left: w305 -> [w343]
              tunnel: w309 -> [w338]
              tunnel: w311 -> [w341]
              tunnel: w301 -> [w339]
              tunnel: w310 -> [w334]
              shift-right: [w325] -> _
              shift-left: _ -> [w330]
              shift-right: [w329] -> w300
              shift-left: w299 -> [w328]
              shift-right: [w324] -> w298
              shift-left: w297 -> [w323]
              shift-right: [w322] -> w296
              shift-left: w295 -> [w321]
              tunnel: w294 -> [w318]
              i -> [w337]
              n86 = Less Or Equal?(x=w337, y=w338) -> (x <= y?=w342:bool)
              n87 = case shown="False" w342 {
                tunnel: w341 -> [w354 w382]
                tunnel: w337 -> [w363 w381]
                tunnel: w340 -> [w362 w380]
                tunnel: [w360 w378] -> w333
                tunnel: w339 -> [w361 _]
                tunnel: w338 -> [w356 _]
                tunnel: w337 -> [w359 _]
                frame False {
                  n88 = Multiply(x=w356, y=2) -> (x*y=w355:dbl)
                  n89 = Less Or Equal?(x=w359, y=w355) -> (x <= y?=w357:bool)
                  n90 = case shown="True" w357 {
                    tunnel: w363 -> [w370 w377]
                    tunnel: w362 -> [w368 w375]
                    tunnel: w361 -> [_ w373]
                    tunnel: [w366 w372] -> w360
                    tunnel: w356 -> [_ w371]
                    tunnel: w355 -> [w365 _]
                    tunnel: w354 -> [w364 _]
                    frame False {
                      n91 = Subtract(x=w370, y=w365) -> (x-y=w369:dbl)
                      n92 = Multiply(x=w368, y=w369) -> (x*y=w367:dbl)
                      n93 = Add(x=w364, y=w367) -> (x+y=w366:dbl)
                    }
                    frame True {
                      n94 = Subtract(x=w377, y=w371) -> (x-y=w376:dbl)
                      n95 = Multiply(x=w375, y=w376) -> (x*y=w374:dbl)
                      n96 = Subtract(x=w373, y=w374) -> (x-y=w372:dbl)
                    }
                  }
                }
                frame True {
                  n97 = Multiply(x=w380, y=w381) -> (x*y=w379:dbl)
                  n98 = Add(x=w382, y=w379) -> (x+y=w378:dbl)
                }
              }
              n99 = Absolute Value(x=w333) -> (abs(x)=w332:dbl)
              n100 = stacked-sequence {
                tunnel: w344 -> [w383 _ _]
                tunnel: w332 -> [w384 _ w457]
                tunnel: w343 -> [_ _ w460]
                tunnel: [_ _ w459] -> w326
                tunnel: [_ _ w458] -> w336
                tunnel: [_ _ w457] -> w335
                tunnel: [_ _ w456] -> w325
                tunnel: w330 -> [_ _ w455]
                tunnel: [_ _ w454] -> w331
                tunnel: [_ _ w453] -> w329
                tunnel: w328 -> [_ _ w446]
                tunnel: [_ _ w452] -> w324
                tunnel: w323 -> [_ _ w447]
                tunnel: [_ _ w451] -> w322
                tunnel: w321 -> [_ _ w450]
                tunnel: [_ _ w449] -> w320
                tunnel: [_ _ w448] -> w319
                tunnel: w318 -> [_ _ w396]
                frame #0 {
                  n101 = Format Into String(format string="SLVLD1,%.3f;", w384) -> (resulting string=w390:string)  [unwired: 2 in, 1 out]
                  n102 = Format Into String(format string="SLVLD2,%.3f;", w384) -> (resulting string=w387:string)  [unwired: 2 in, 1 out]
                  n103 = Concatenate Strings(w390, "\r") -> (w389:string)
                  n104 = Concatenate Strings(w387, "\r") -> (w386:string)
                  n105 = VISA Write(VISA resource name=w383, write buffer=w389) -> ()  [unwired: 1 in, 3 out]
                  n106 = VISA Write(VISA resource name=w383, write buffer=w386) -> ()  [unwired: 1 in, 3 out]
                  "Sine voltage" <- w384
                }
                frame #1 {
                  n107 = Multiply(x="lockin waiting (s)", y=1000) -> (x*y=w395:dbl)
                  n108 = Wait (ms)(milliseconds to wait=w395) -> ()  [unwired: 1 out]
                }
                frame #2 {
                  n109 = flat-sequence {
                    tunnel: w460 -> [w488]
                    tunnel: w457 -> [w487]
                    tunnel: w455 -> [w486]
                    tunnel: w450 -> [w480]
                    tunnel: [w484] -> w445
                    tunnel: [w476] -> w443
                    tunnel: [w477] -> w441
                    tunnel: [w474] -> w439
                    tunnel: [w477] -> w437
                    tunnel: [w477] -> w435
                    tunnel: [w477] -> w433
                    tunnel: [w477] -> w431
                    tunnel: [w476] -> w429
                    tunnel: [w475] -> w427
                    tunnel: [w474] -> w425
                    tunnel: [w473] -> w423
                    tunnel: ["Clear Plot B"] -> w421
                    tunnel: ["Clear Plot A"] -> w419
                    tunnel: [w464] -> w417
                    tunnel: [w466] -> w415
                    tunnel: [w465] -> w413
                    tunnel: [w470] -> w411
                    tunnel: [w469] -> w409
                    tunnel: w396 -> [w461]
                    tunnel: w445 -> [w510]
                    tunnel: [w510] -> w444
                    tunnel: w443 -> [w509]
                    tunnel: [w509] -> w442
                    tunnel: w441 -> [w508]
                    tunnel: [w508] -> w440
                    tunnel: w439 -> [w507]
                    tunnel: [w507] -> w438
                    tunnel: w437 -> [w506]
                    tunnel: [w506] -> w436
                    tunnel: w435 -> [w505]
                    tunnel: [w505] -> w434
                    tunnel: w433 -> [w504]
                    tunnel: [w504] -> w432
                    tunnel: w431 -> [w503]
                    tunnel: [w503] -> w430
                    tunnel: w429 -> [w502]
                    tunnel: [w502] -> w428
                    tunnel: w427 -> [w501]
                    tunnel: [w501] -> w426
                    tunnel: w425 -> [w500]
                    tunnel: [w500] -> w424
                    tunnel: w423 -> [w499]
                    tunnel: [w499] -> w422
                    tunnel: w421 -> [w498]
                    tunnel: [w498] -> w420
                    tunnel: w419 -> [w497]
                    tunnel: [w497] -> w418
                    tunnel: w417 -> [w496]
                    tunnel: [w496] -> w416
                    tunnel: w415 -> [w495]
                    tunnel: [w495] -> w414
                    tunnel: w413 -> [w494]
                    tunnel: [w494] -> w412
                    tunnel: w411 -> [w493]
                    tunnel: [w493] -> w410
                    tunnel: w409 -> [w492]
                    tunnel: [w492] -> w408
                    tunnel: w444 -> [w514]
                    tunnel: w442 -> [w548]
                    tunnel: w440 -> [w547]
                    tunnel: w438 -> [w546]
                    tunnel: w436 -> [w545]
                    tunnel: w434 -> [w543]
                    tunnel: w432 -> [w541]
                    tunnel: w430 -> [w539]
                    tunnel: w428 -> [w536]
                    tunnel: w426 -> [w535]
                    tunnel: w424 -> [w532]
                    tunnel: w422 -> [w531]
                    tunnel: w447 -> [w529]
                    tunnel: w420 -> [w528]
                    tunnel: w446 -> [w526]
                    tunnel: w418 -> [w525]
                    tunnel: w416 -> [w521]
                    tunnel: w414 -> [w520]
                    tunnel: w412 -> [w519]
                    tunnel: w410 -> [w516]
                    tunnel: w408 -> [w515]
                    tunnel: [w514] -> w407
                    tunnel: [w534] -> w406
                    tunnel: [w548] -> w405
                    tunnel: [w547] -> w404
                    tunnel: [w512] -> w403
                    tunnel: [w513] -> w402
                    tunnel: [w537] -> w401
                    tunnel: [w533] -> w400
                    tunnel: [w530] -> w399
                    tunnel: [w546] -> w398
                    tunnel: [w518] -> w397
                    tunnel: [w550] -> w448
                    tunnel: [w551] -> w449
                    tunnel: [w552] -> w451
                    tunnel: [w553] -> w452
                    tunnel: [w554] -> w453
                    tunnel: [w555] -> _
                    tunnel: [w556] -> w454
                    tunnel: [w557] -> w456
                    tunnel: [w558] -> w458
                    tunnel: [w559] -> w459
                    tunnel: [w560] -> _
                    tunnel: w407 -> [w560]
                    tunnel: w406 -> [w559]
                    tunnel: w405 -> [w558]
                    tunnel: w404 -> [w557]
                    tunnel: w403 -> [w556]
                    tunnel: w402 -> [w555]
                    tunnel: w401 -> [w554]
                    tunnel: w400 -> [w553]
                    tunnel: w399 -> [w552]
                    tunnel: w398 -> [w551]
                    tunnel: w397 -> [w550]
                    frame #0 {
                      w466 = u8 1 items=["Channel A", "Channel B"] ("Channel A/B for Parameter1")
                      w469 = u8 0 items=["Channel A", "Channel B"] ("Channel A/B for Parameter1")
                      n110 = Format Into String(0) -> (error out=w485:errorcluster)  [unwired: 3 in, 1 out]
                      n111 = Format Into String(0) -> (error out=w467:errorcluster)  [unwired: 3 in, 1 out]
                      n112 = call <instrlib>:"OE1022D_Read 1 parameter_mean.vi"("错误输入（无错误）"=w485, "Parameter"="Parameter A", "Channel (0: A)"=w469, "VISA resource name"=w461) -> ("error out"=w470:errorcluster, "Measurement"=w478:dbl, "VISA resource name out"=w484:refnum<visa-resource-name>)  [unwired: 5 in]
                      n113 = call <instrlib>:"OE1022D_Read 1 parameter_mean.vi"("Parameter 2"="Parameter B", "错误输入（无错误）"=w467, "Channel (0: A)"=w466, "VISA resource name"=w461) -> ("error out"=w464:errorcluster, "Measurement"=w463:dbl, "VISA resource name out"=w465:refnum<visa-resource-name>)  [unwired: 5 in]
                      n114 = Multiply(x=w478, y=1000000.0) -> (x*y=w476:dbl)
                      "para1 Measurement" <- w476
                      n115 = Multiply(x=w463, y=1000000.0) -> (x*y=w474:dbl)
                      "para2 Measurement" <- w474
                      n116 = Build Array(w474) -> (w481:dbl[])
                      n117 = Build Array(w476) -> (w489:dbl[])
                      n118 = Select(t=w481, s="Clear Plot B", f=w480) -> (s? t:f=w473:dbl[])
                      n119 = Select(t=w489, s="Clear Plot A", f=w488) -> (s? t:f=w475:dbl[])
                      n120 = Build Array (concatenate)(w487, w486) -> (w477:dbl[])
                    }
                    frame #1 {
                      n121 = Wait (ms)(milliseconds to wait=u32 50) -> ()  [unwired: 1 out]
                    }
                    frame #2 {
                      n122 = Build Array (concatenate)(w532, w531) -> (w530:dbl[])
                      n123 = Build Array (concatenate)(w536, w535) -> (w534:dbl[])
                      n124 = call <instrlib>:"OE1022D_Read 1 parameter_mean.vi"("错误输入（无错误）"=w516, "Parameter"="Phase A", "Channel (0: A)"=w515, "VISA resource name"=w514) -> ("error out"=w513:errorcluster, "Measurement"=w512:dbl)  [unwired: 5 in, 1 out]
                      "phase A" <- w512
                      n125 = Bundle(w543, w530) -> (→"XY Graph 3":cluster{dbl[], dbl[]})  [unwired: 1 in]
                      n126 = call <instrlib>:"OE1022D_Read 1 parameter_mean.vi"("Parameter 2"="Phase B", "错误输入（无错误）"=w521, "Channel (0: A)"=w520, "VISA resource name"=w519) -> ("Measurement"=w518:dbl)  [unwired: 5 in, 2 out]
                      "phase B" <- w518
                      n127 = Bundle(w541, w534) -> (→"XY Graph":cluster{dbl[], dbl[]})  [unwired: 1 in]
                      n128 = Build Array(w512) -> (w522:dbl[])
                      n129 = Build Array(w518) -> (w523:dbl[])
                      n130 = Select(t=w522, s=w525, f=w526) -> (s? t:f=w524:dbl[])
                      n131 = Select(t=w523, s=w528, f=w529) -> (s? t:f=w527:dbl[])
                      n132 = Build Array (concatenate)(w512, w524) -> (w537:dbl[])
                      n133 = Build Array (concatenate)(w518, w527) -> (w533:dbl[])
                      n134 = Bundle(w539, w537) -> (→"XY Graph 2":cluster{dbl[], dbl[]})  [unwired: 1 in]
                      n135 = Bundle(w545, w533) -> (→"XY Graph 4":cluster{dbl[], dbl[]})  [unwired: 1 in]
                    }
                    frame #3 {
                      n136 = Wait (ms)(milliseconds to wait=u32 50) -> ()  [unwired: 1 out]
                    }
                  }
                }
              }
              n137 = case shown="True" "Save data or not" {
                tunnel: w336 -> [_ w348]
                tunnel: w335 -> [_ w353]
                tunnel: w334 -> [_ w351]
                tunnel: w331 -> [_ w347]
                tunnel: w320 -> [_ w346]
                tunnel: w319 -> [_ w345]
                frame False {
                }
                frame True {
                  n138 = Build Array(w353, w348, w347, w346, w345) -> (w350:dbl[])
                  n139 = call-poly <vilib>:"Write Delimited Spreadsheet.vi"("file path (dialog if empty)"=w351, "format (%.3f)"="%.10f", "1D data"=w350, "append to file? (new file:F)"=TRUE) -> ()  [unwired: 10 in, 2 out]
                }
              }
            }
          }
        }
      }
    }
  }
  n140 = Format Into String(initial string="path (folder + filename)", w2, "Hz", "Series Resistance", w6, "K", w10, "Oe", ".txt") -> (resulting string=w7:string)  [unwired: 2 in, 1 out]
  n141 = String To Path(string=w7) -> (path=w13:path)
